vi "Serial_Read_ALL.vi"(6 "Error IN":errorcluster, 9 "Visa Resource IN":refnum<visa-resource-name>="MULTIMEK") -> (0 "Error OUT":errorcluster, 2 "String":string, 3 "Visa Resource OUT":refnum<visa-resource-name>)   [LabVIEW 2013]
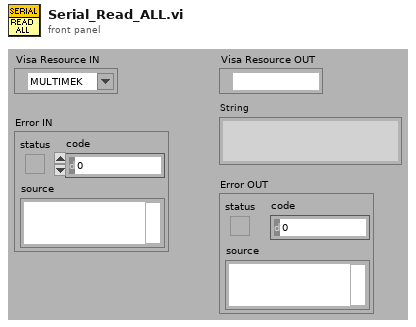
[diagram p1: front panel]
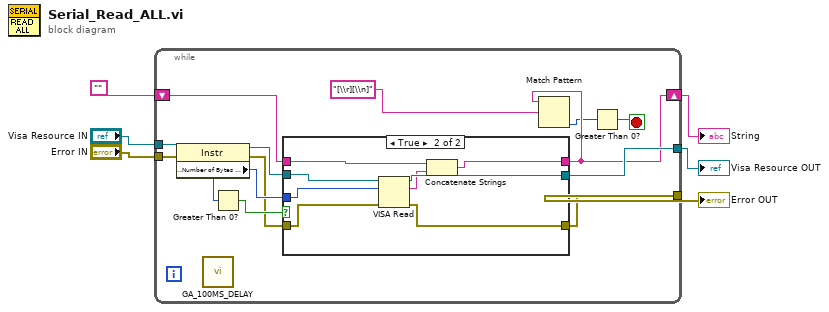
[diagram p0: block diagram]
diagram:
  n1 = while {
    tunnel: "Visa Resource IN" -> [w19]
    tunnel: [w17] -> w2
    tunnel: "Error IN" -> [w13]
    tunnel: [w12] -> w3
    shift-right: [w10] -> w6
    shift-left: "" -> [w11]
    stop <- w9 stop-if-true
    n2 = property class="Instr"(reference=w19, error in=w13) -> (reference out=w18:refnum<visa-resource-name>, error out=w14:errorcluster, "Serial Settings:Number of Bytes at Serial Port"=w15:u32)
    n3 = call "GA_100MS_DELAY.vi"() -> ()  [unwired: 1 in, 11 out]
    n4 = Greater Than 0?(x=w15) -> (x > 0?=w16:bool)
    n5 = case shown="True" w16 {
      tunnel: w18 -> [w22 w30]
      tunnel: [w22 w29] -> w17
      tunnel: w15 -> [_ w28]
      tunnel: w14 -> [w21 w27]
      tunnel: [w21 w26] -> w12
      tunnel: w11 -> [w20 w25]
      tunnel: [w20 w23] -> w10
      frame False {
      }
      frame True {
        n6 = VISA Read(VISA resource name=w30, byte count=w28, error in (no error)=w27) -> (VISA resource name out=w29:refnum<visa-resource-name>, read buffer=w24:string, error out=w26:errorcluster)  [unwired: 1 out]
        n7 = Concatenate Strings(w25, w24) -> (w23:string)
      }
    }
    n8 = Match Pattern(string=w10, regular expression="[\\r][\\n]") -> (offset past match=w8:i32)  [unwired: 4 out]
    n9 = Greater Than 0?(x=w8) -> (x > 0?=w9:bool)
  }
  "String" <- w6
  "Error OUT" <- w3
  "Visa Resource OUT" <- w2
